vi "Creating Folder.vi"(11 "Input String Path":string) -> (3 "Output String Path":string)   [LabVIEW 2011]
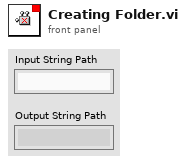
[diagram p1: front panel]
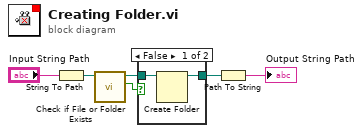
[diagram p0: block diagram]
diagram:
  n1 = String To Path(string="Input String Path") -> (path=w6:path)
  n2 = call <vilib>:"Check if File or Folder Exists.vi"("path"=w6) -> ("file or folder exists?"=w4:bool, "dup path"=w3:path)  [unwired: 8 in, 1 out]
  n3 = case shown="False" w4 {
    tunnel: [w8 w9] -> w5
    tunnel: w3 -> [w7 w9]
    frame False {
      n4 = Create Folder(path (use dialog)=w7) -> (created path=w8:path)  [unwired: 2 in, 2 out]
    }
    frame True {
    }
  }
  n5 = Path To String(path=w5) -> (string=→"Output String Path":string)
